vi "温湿度采集.vi"(11 "Modbus Master输入":refnum<class "Modbus Master.lvclass">) -> (1 "温度":string, 3 "湿度":string)   [LabVIEW 2015]
uses:
  <vilib>/NI/Modbus Library/API/Master/Modbus Master.lvclass
panel:
  out "湿度":dbl
  out "温度":dbl
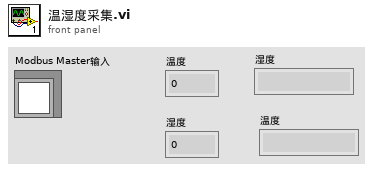
[diagram p1: front panel]
types:
  T1 = cluster{"地址":u16, "数量":u16, "寄存器值":u16[], "名称":string}[]
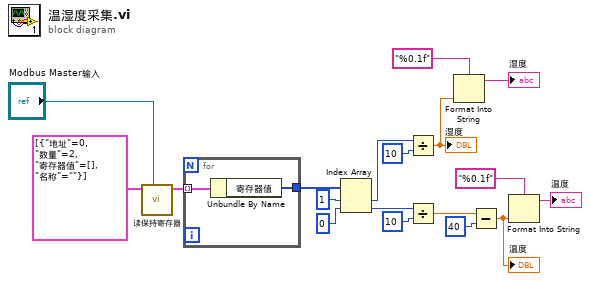
[diagram p0: block diagram]
diagram:
  n1 = call "读保持寄存器.vi"("MB_实体"="Modbus Master输入", "读保持寄存器信息组__输入"=T1 [{"地址"=0, "数量"=2, "寄存器值"=[], "名称"=""}]) -> ("读保持寄存器信息组_输出"=w11:T1)  [unwired: 7 in, 2 out]
  n2 = for {
    tunnel: w11 -> [w20] mode=indexing
    tunnel: [w19] -> w14
    n3 = Unbundle By Name(w20) -> ("寄存器值"=w19:u16[])
  }
  n4 = Index Array(array=w14, index #1=1 ("索引"), index #2=0 ("索引")) -> (element #1=w2:u16, element #2=w1:u16)
  n5 = Divide(x=w2, y=u32 10) -> (x/y=w7:dbl)
  "湿度" <- w7
  n6 = Divide(x=w1, y=u32 10) -> (x/y=w16:dbl)
  n7 = Format Into String(format string="%0.1f" ("格式字符串"), w7) -> (resulting string=→"湿度":string)  [unwired: 2 in, 1 out]
  n8 = Subtract(x=w16, y=u32 40) -> (x-y=w5:dbl)
  "温度" <- w5
  n9 = Format Into String(format string="%0.1f" ("格式字符串"), w5) -> (resulting string=→"温度":string)  [unwired: 2 in, 1 out]
